vi "CalculerPolynome.vi"(6 "Résidu [in]":dbl, 9 "Meilleure poly [in]":dbl[](array[numeric]), 10 "Y":dbl[](array[numeric]), 11 "X":dbl[](array[numeric])) -> (2 "Résidu [out]":dbl, 3 "Meilleur poly [out]":dbl[](array[numeric]))   [LabVIEW 2013]
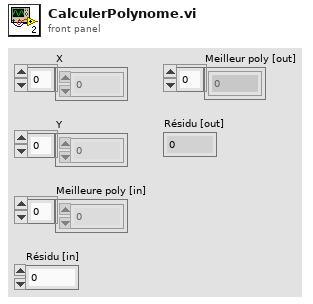
[diagram p1: front panel]
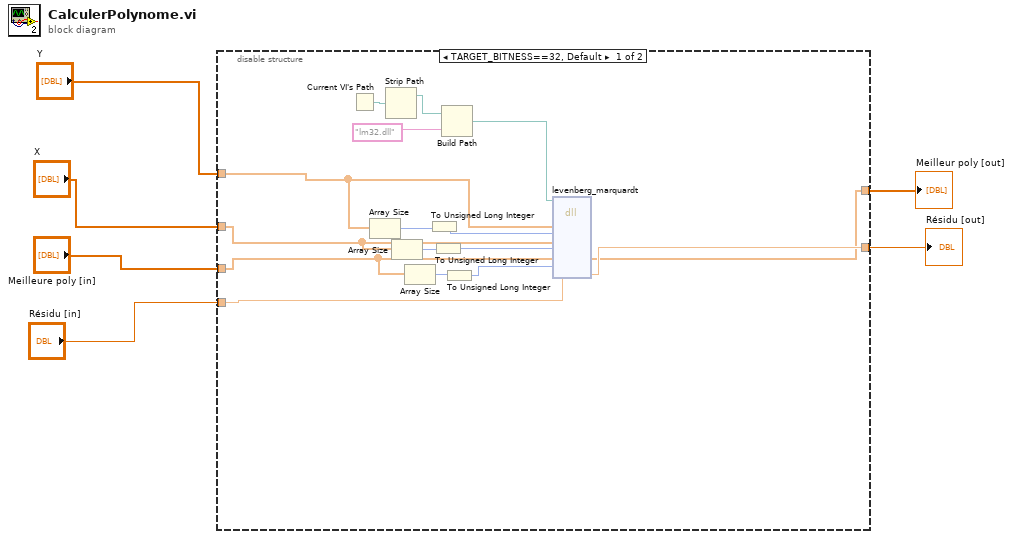
[diagram p0: block diagram]
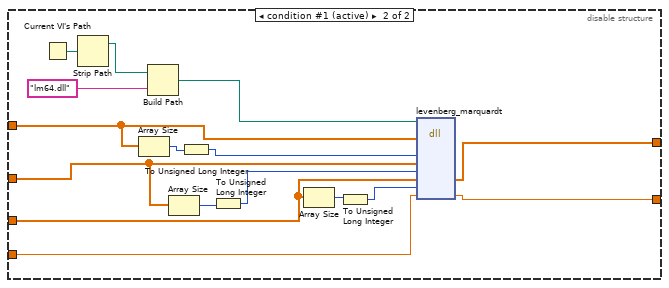
[diagram p2: hidden frame]
diagram:
  n1 = disable-structure shown="TARGET_BITNESS==32, Default" {
    disable-tunnel: "X" -> [w9 w34]
    disable-tunnel: "Y" -> [w12 w33]
    disable-tunnel: "Meilleure poly [in]" -> [w15 w28]
    disable-tunnel: "Résidu [in]" -> [w18 w25]
    disable-tunnel: [w8 w24] -> w5
    disable-tunnel: [w7 w23] -> w6
    frame condition #0 {
      n2 = Current VI's Path() -> (path=w22:path)
      n3 = Array Size(array=w12) -> (size(s)=w13:i32)
      n4 = Strip Path(path=w22) -> (stripped path=w21:path)  [unwired: 1 out]
      n5 = Array Size(array=w9) -> (size(s)=w10:i32)
      n6 = Array Size(array=w15) -> (size(s)=w16:i32)
      n7 = To Unsigned Long Integer(number=w13) -> (unsigned 32bit integer=w14:u32)
      n8 = To Unsigned Long Integer(number=w10) -> (unsigned 32bit integer=w11:u32)
      n9 = Build Path(base path=w21, name or relative path="lm32.dll") -> (appended path=w19:path)
      n10 = To Unsigned Long Integer(number=w16) -> (unsigned 32bit integer=w17:u32)
      n11 = dll-call lib="?" fn="levenberg_marquardt"(path in=w19, "yobs"=w12, "yobslength"=w14, "xobs"=w9, "xobslength"=w11, "polyptr"=w15, "numCoeffs"=w17, "e"=w18) -> ("polyptr"=w7:dbl[], "e"=w8:dbl)  [unwired: 8 in, 2 out]
    }
    frame condition #1 (active) {
      n12 = Current VI's Path() -> (path=w38:path)
      n13 = Strip Path(path=w38) -> (stripped path=w37:path)  [unwired: 1 out]
      n14 = Array Size(array=w33) -> (size(s)=w30:i32)
      n15 = Build Path(base path=w37, name or relative path="lm64.dll") -> (appended path=w35:path)
      n16 = Array Size(array=w34) -> (size(s)=w32:i32)
      n17 = To Unsigned Long Integer(number=w30) -> (unsigned 32bit integer=w29:u32)
      n18 = To Unsigned Long Integer(number=w32) -> (unsigned 32bit integer=w31:u32)
      n19 = Array Size(array=w28) -> (size(s)=w27:i32)
      n20 = To Unsigned Long Integer(number=w27) -> (unsigned 32bit integer=w26:u32)
      n21 = dll-call lib="?" fn="levenberg_marquardt"(path in=w35, "yobs"=w33, "yobslength"=w29, "xobs"=w34, "xobslength"=w31, "polyptr"=w28, "numCoeffs"=w26, "e"=w25) -> ("polyptr"=w23:dbl[], "e"=w24:dbl)  [unwired: 8 in, 2 out]
    }
  }
  "Meilleur poly [out]" <- w6
  "Résidu [out]" <- w5
